vi "Enable_AFR_EGT_Graph (SubVI).vi"(0 "Leistungsgraph":refnum<vi>, 1 "AFR EGT":bool, 2 "Y-Koord. Graph-Reset-Button (782)":i32, 3 "Lambda":refnum<vi>, 5 "Reset Skalierung":refnum<vi>, 7 "Höhe Leistungs-Graph":u32, 9 "AFR EGT Gaph":refnum<vi>, 11 "Auto Skalierung":refnum<vi>, 12 "AFR":refnum<vi>, 13 "EGT [°C]":refnum<vi>, 14 "Skalierungsfaktor Leistungsgraph":dbl) -> ()   [LabVIEW 2014]
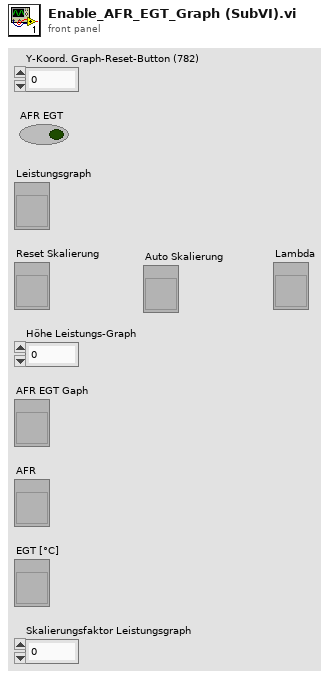
[diagram p1: front panel]
types:
  T1 = typedef "LVRangeTypeDef.ctl" = cluster{"Minimum":dbl, "Maximum":dbl, "Increment":dbl, "Minor Increment":dbl, "Start":dbl}
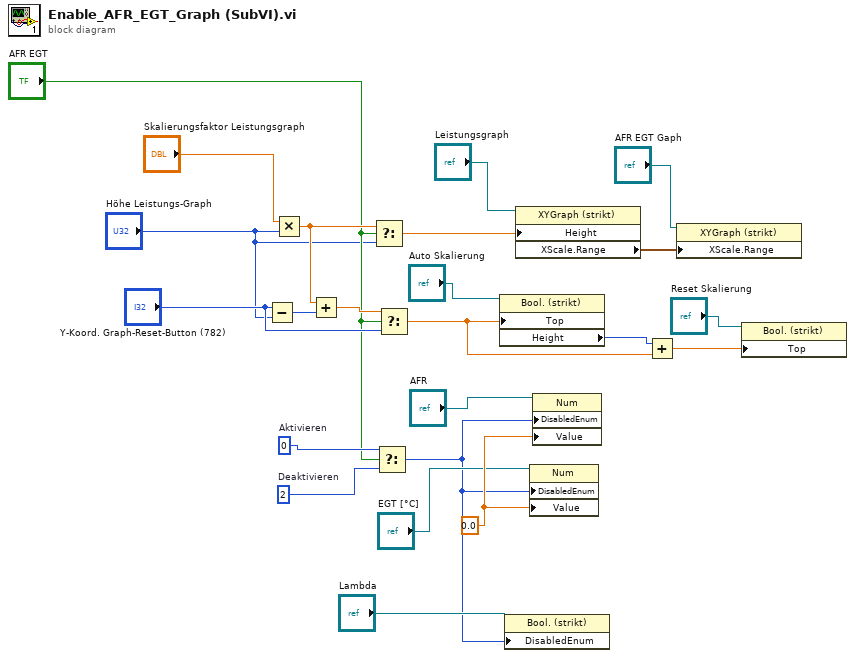
[diagram p0: block diagram]
diagram:
  w23 = 0  # Aktivieren
  w13 = 0.0
  w18 = 2  # Deaktivieren
  n1 = Subtract(x="Y-Koord. Graph-Reset-Button (782)", y="Höhe Leistungs-Graph") -> (x-y=w19:u32)
  n2 = Multiply(x="Skalierungsfaktor Leistungsgraph", y="Höhe Leistungs-Graph") -> (x*y=w20:dbl)
  n3 = Add(x=w20, y=w19) -> (x+y=w21:dbl)
  n4 = Select(t=w20, s="AFR EGT", f="Höhe Leistungs-Graph") -> (s? t:f=w15:dbl)
  n5 = Select(t=w23, s="AFR EGT", f=w18) -> (s? t:f=w6:i32)
  n6 = Select(t=w21, s="AFR EGT", f="Y-Koord. Graph-Reset-Button (782)") -> (s? t:f=w3:dbl)
  n7 = property on="Eigenschaftsknoten" class="Bool. (strikt)"(reference="Auto Skalierung", "Top"=w3) -> ("Height"=w4:u32)  [unwired: 1 in, 2 out]
  n8 = property on="Eigenschaftsknoten" class="Bool. (strikt)"(reference="Lambda", "DisabledEnum"=w6) -> ()  [unwired: 1 in, 2 out]
  n9 = property on="Eigenschaftsknoten" class="XYGraph (strikt)"(reference="Leistungsgraph", "Height"=w15) -> ("XScale.Range"=w12:T1)  [unwired: 1 in, 2 out]
  n10 = property on="Eigenschaftsknoten" class="Num"(reference="EGT [°C]", "DisabledEnum"=w6, "Value"=w13) -> ()  [unwired: 1 in, 2 out]
  n11 = property on="Eigenschaftsknoten" class="Num"(reference="AFR", "DisabledEnum"=w6, "Value"=w13) -> ()  [unwired: 1 in, 2 out]
  n12 = Add(x=w4, y=w3) -> (x+y=w1:dbl)
  n13 = property on="Eigenschaftsknoten" class="XYGraph (strikt)"(reference="AFR EGT Gaph", "XScale.Range"=w12) -> ()  [unwired: 1 in, 2 out]
  n14 = property on="Eigenschaftsknoten" class="Bool. (strikt)"(reference="Reset Skalierung", "Top"=w1) -> ()  [unwired: 1 in, 2 out]
